vi "Initialize and Home SubVi.vi"() -> (0 "error out":errorcluster, 1 "reference out":refnum<k24>)   [LabVIEW 2017]
uses:
  Newport.XPS.CommandInterface
  Initialize and Home Enum.ctl
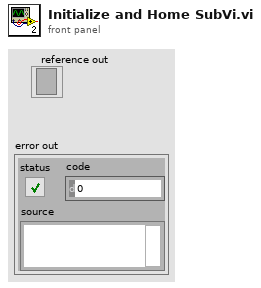
[diagram p1: front panel]
types:
  T1 = typedef "Initialize and Home Enum.ctl" = enum16{"Initialize", "Search Home", "Stop Command"}
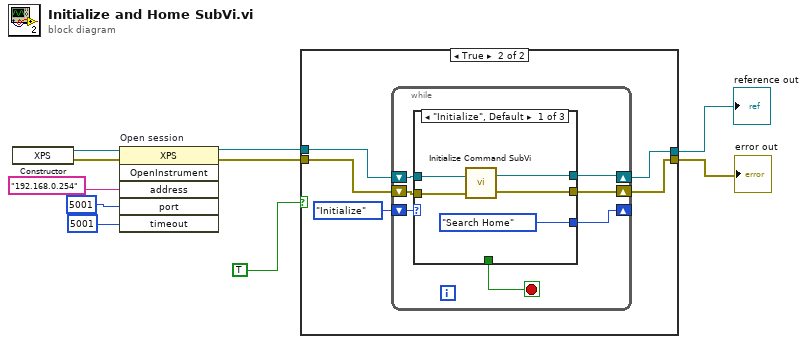
[diagram p0: block diagram]
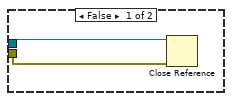
[diagram p2: hidden frame]
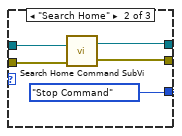
[diagram p3: hidden frame]
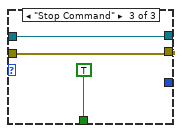
[diagram p4: hidden frame]
diagram:
  n1 = constructor class="XPS"() -> (reference out=w6:refnum<k24>, error out=w7:errorcluster)  [unwired: 3 in, 1 out]
  n2 = invoke on="Open session" class="XPS" method="OpenInstrument"(reference=w6, error in=w7, "address"="192.168.0.254", "port"=5001, "timeout"=5001) -> (reference out=w2:refnum<k24>, error out=w1:errorcluster)  [unwired: 1 in, 4 out]
  n3 = case shown="True" TRUE {
    tunnel: w2 -> [w12 w16]
    tunnel: w1 -> [w11 w15]
    tunnel: [_ w14] -> w8
    tunnel: [_ w13] -> w9
    frame False {
      n4 = Close Reference(reference=w12, error in (no error)=w11) -> ()  [unwired: 1 out]
    }
    frame True {
      n5 = while {
        shift-right: [w18] -> _
        shift-left: Initialize_and_Home_Enum."Initialize" -> [w24]
        shift-right: [w21] -> w14
        shift-left: w16 -> [w23]
        shift-right: [w20] -> w13
        shift-left: w15 -> [w22]
        stop <- w19 stop-if-true
        n6 = case shown="\"Initialize\", Default" w24 {
          tunnel: w23 -> [w28 w33 w36]
          tunnel: w22 -> [w27 w32 w35]
          tunnel: [w26 w31 w36] -> w21
          tunnel: [w25 w30 w35] -> w20
          tunnel: [_ _ TRUE] -> w19
          tunnel: [Initialize_and_Home_Enum."Search Home" Initialize_and_Home_Enum."Stop Command" _] -> w18
          frame "Initialize", Default {
            n7 = call "Initialize Command SubVi.vi"("error in"=w27, "reference in"=w28) -> ("error out"=w25:errorcluster, "reference out"=w26:refnum<k24>)
          }
          frame "Search Home" {
            n8 = call "Search Home Command SubVi.vi"("error in"=w32, "reference in"=w33) -> ("error out"=w30:errorcluster, "reference out"=w31:refnum<k24>)
          }
          frame "Stop Command" {
          }
        }
      }
    }
  }
  "error out" <- w9
  "reference out" <- w8
